vi "Teleop.vi"(10 "Match Info":T1={"Autonomous Elapsed Seconds"=0.0, "TeleOp Elapsed Seconds"=0.0, "Disabled Elapsed Seconds"=0.0, "Visited Autonomous"=FALSE, "Visited TeleOp"=FALSE, "Visited Disabled"=FALSE, "Autonomous Settings"={"Autonomous Style"=enum."Independent", "VI Refnum"=refnum}}, 11 "Call Context":T2) -> ()   [LabVIEW 2013]
doc: "This VI is called for each TeleOp packet received from the DS where the robot is not disabled. It is often used to read from the joysticks and update I/O or to update setpoints for timed control loops. It should complete and return within 20 milliseconds or it may miss DS packets."
uses:
  <vilib>/Rock Robotics/WPI/DriverStation/WPI_DriverStationDerivedRobotMode.ctl
  <vilib>/Rock Robotics/WPI/DriverStation/WPI_DriverStationMatch Info.ctl
  Robot Global Data.vi
  <vilib>/Rock Robotics/WPI/Joystick/WPI_JoystickGetSetRefNum.vi
panel:
  in  "HarvSpeed":dbl=0.5
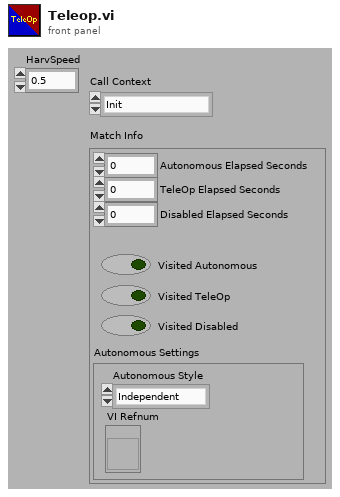
[diagram p1: front panel]
types:
  T1 = typedef "WPI_DriverStationMatch Info.ctl" = cluster{"Autonomous Elapsed Seconds":dbl, "TeleOp Elapsed Seconds":dbl, "Disabled Elapsed Seconds":dbl, "Visited Autonomous":bool, "Visited TeleOp":bool, "Visited Disabled":bool, "Autonomous Settings":cluster{"Autonomous Style":enum16{"Iterative", "Independent"}, "VI Refnum":refnum<vi>}}
  T2 = typedef "WPI_DriverStationDerivedRobotMode.ctl" = enum16{"Init", "Execute", "Stop"}
  T3 = typedef "WPI_JoystickDevRef.ctl" = cluster{"Device":T4}
  T4 = typedef "WPI_JoystickDeviceEnum.ctl" = enum16{"USB 1", "USB 2", "USB 3", "USB 4", "Kinect 1", "Kinect 2"}
  T5 = cluster{"axis 1 (x)":dbl, "axis 2 (y)":dbl, "axis 3 (throttle)":dbl, "axis 4":dbl, "axis 5":dbl, "axis 6":dbl}
  T6 = typedef "WPI_MotorControlDeviceRef.ctl" = cluster{"DeviceStatus":errorcluster, "Type":enum16{"PWM", "CAN"}, "PWM":cluster{"Digital Module":T7, "PWM Channel":T8, "DeadBand":T9}, "CAN":cluster{"Device Number":u8, "Control Mode":T10, "Semaphore":T11, "Max Vout":dbl}, "Invert":bool, "TransformRef":T12, "InvTransformRef":T12}
  T7 = typedef "FPGA_TypedefDigitalModule.ctl" = enum16{"Digital Module 1", "Digital Module 2"}
  T8 = typedef "FPGA_DIOPWMChannel.ctl" = enum8{"PWM 1", "PWM 2", "PWM 3", "PWM 4", "PWM 5", "PWM 6", "PWM 7", "PWM 8", "PWM 9", "PWM 10", "Invalid"}
  T9 = typedef "WPI_PWMDeadband.ctl" = cluster{"Name":string, "maxPositivePwm":i32, "minPositivePwm":i32, "centerPwm":i32, "maxNegativePwm":i32, "minNegativePwm":i32, "angularRange":u16}
  T10 = typedef "WPI_CANJaguar_ControlMode.ctl" = enum8{"Percent VBus", "Current", "Speed", "Position", "Voltage"}
  T11 = typedef "Semaphore RefNum" = refnum<k1>
  T12 = typedef "WPI_PWMTransform_ConPane.ctl" = refnum<vi>
  T13 = cluster{"Driver Station Digital Input (1-8)[0]":bool, "Driver Station Digital Input (1-8)[1]":bool, "Driver Station Digital Input (1-8)[2]":bool, "Driver Station Digital Input (1-8)[3]":bool, "Driver Station Digital Input (1-8)[4]":bool, "Driver Station Digital Input (1-8)[5]":bool, "Driver Station Digital Input (1-8)[6]":bool, "Driver Station Digital Input (1-8)[7]":bool, "Driver Station Digital Input (1-8)[8]":bool}
  T14 = typedef "WPI_JoystickButtonState.ctl" = cluster{"Button 1":bool, "Button 2":bool, "Button 3":bool, "Button 4":bool, "Button 5":bool, "Button 6":bool, "Button 7":bool, "Button 8":bool, "Button 9":bool, "Button 10":bool, "Button 11":bool, "Button 12":bool}
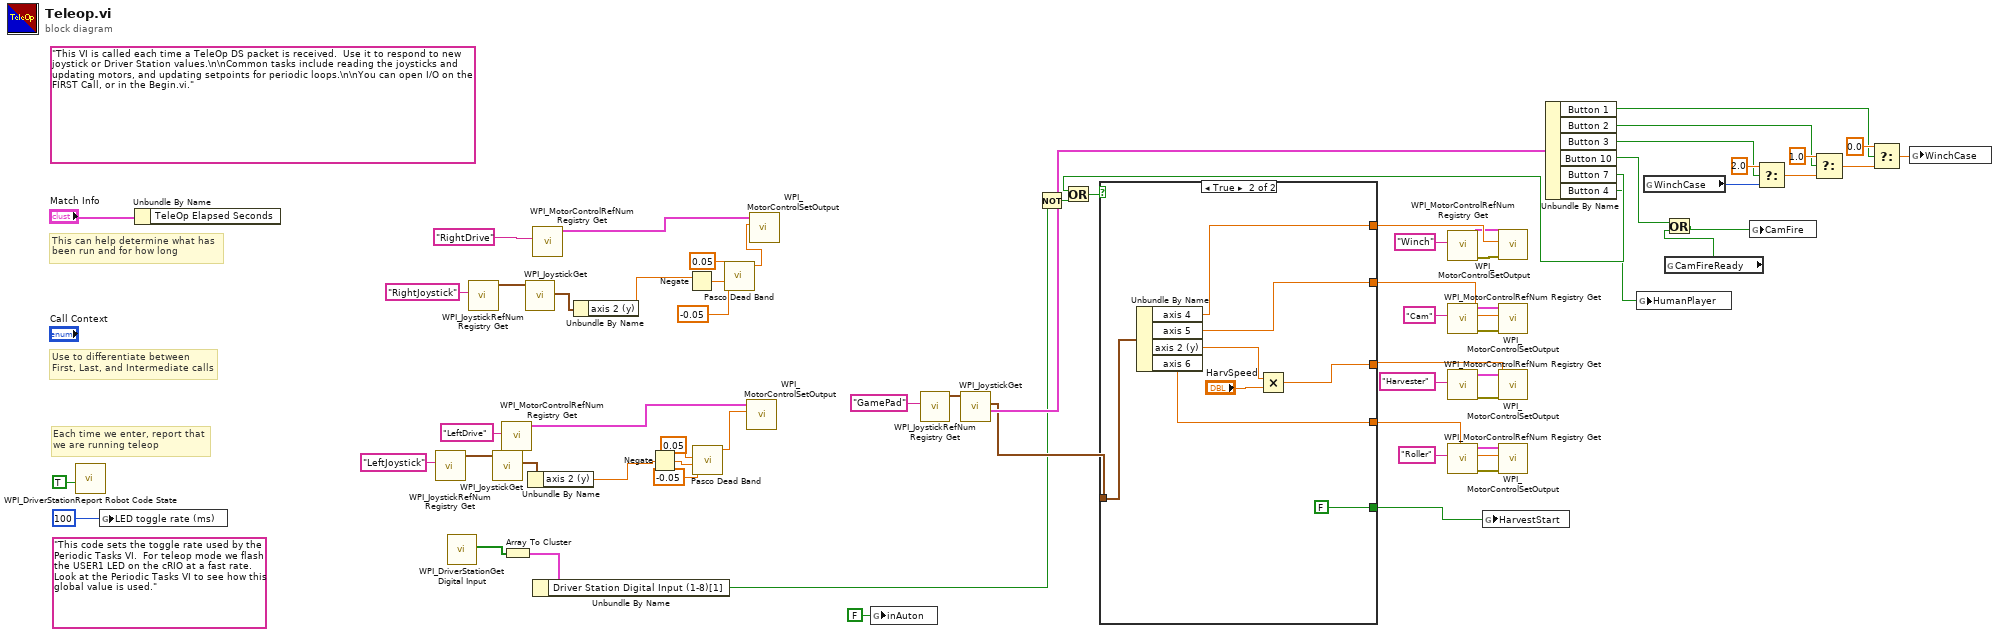
[diagram p0: block diagram]
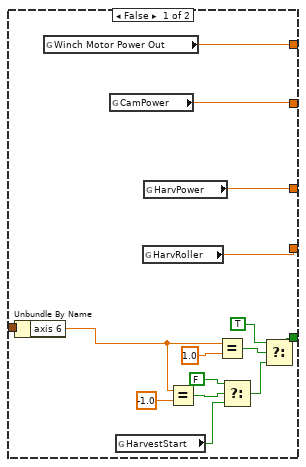
[diagram p2: hidden frame]
diagram:
  (unwired) "This code sets the toggle rate used by the Periodic Tasks VI.  For teleop mode we flash the USER1 LED on the cRIO at a fast rate.  Look at the Periodic Tasks VI to see how this global value is used."
  (unwired) "This VI is called each time a TeleOp DS packet is received.  Use it to respond to new joystick or Driver Station values.\n\nCommon tasks include reading the joysticks and updating motors, and updating setpoints for periodic loops.\n\nYou can open I/O on the FIRST Call, or in the Begin.vi."
  # "Each time we enter, report that\nwe are running teleop"
  # "Use to differentiate between\nFirst, Last, and Intermediate calls"
  # "This can help determine what has\nbeen run and for how long"
  n1 = call <vilib>:"WPI_DriverStationReport Robot Code State.vi"("TeleOp"=TRUE ("Autonomous")) -> ()  [unwired: 10 in, 1 out]
  n2 = global write "Robot Global Data.vi" "LED toggle rate (ms)"(u32 100 ("LED ms toggle rate")) -> ()
  n3 = Unbundle By Name("Match Info") -> ()  [unwired: 1 out]
  n4 = call <vilib>:"WPI_JoystickRefNum Registry Get.vi"("refnum name"="LeftJoystick") -> ("JoystickDevRef"=w54:T3)  [unwired: 9 in, 1 out]
  n5 = call <vilib>:"WPI_DriverStationGet Digital Input.vi"() -> ("Driver Station Digital Input (1-8)"=w9:bool[])  [unwired: 11 in]
  n6 = call <vilib>:"WPI_JoystickRefNum Registry Get.vi"("refnum name"="RightJoystick") -> ("JoystickDevRef"=w59:T3)  [unwired: 9 in, 1 out]
  n7 = call <vilib>:"WPI_JoystickGet.vi"("JoystickDevRef"=w54) -> ("Axes"=w53:T5)  [unwired: 4 in, 2 out]
  n8 = call <vilib>:"WPI_MotorControlRefNum Registry Get.vi"("refnum name"="LeftDrive") -> ("MotorControlDevRef"=w57:T6)  [unwired: 9 in, 1 out]
  n9 = Array To Cluster(array=w9) -> (cluster=w8:T13)
  n10 = call <vilib>:"WPI_JoystickGet.vi"("JoystickDevRef"=w59) -> ("Axes"=w58:T5)  [unwired: 4 in, 2 out]
  n11 = Unbundle By Name(w53) -> ("axis 2 (y)"=w52:dbl)
  n12 = call <vilib>:"WPI_MotorControlRefNum Registry Get.vi"("refnum name"="RightDrive") -> ("MotorControlDevRef"=w62:T6)  [unwired: 9 in, 1 out]
  n13 = Unbundle By Name(w8) -> ("Driver Station Digital Input (1-8)[1]"=w7:bool)
  n14 = Unbundle By Name(w58) -> ("axis 2 (y)"=w51:dbl)
  n15 = Negate(x=w52) -> (-x=w46:dbl)
  n16 = Negate(x=w51) -> (-x=w50:dbl)
  n17 = call "Pasco Dead Band.vi"("lower limit"=-0.05, "PWM Power"=w46, "upper limit"=0.05) -> ("PWM Power"=w43:dbl)  [unwired: 7 in, 1 out]
  n18 = call "Pasco Dead Band.vi"("lower limit"=-0.05, "PWM Power"=w50, "upper limit"=0.05) -> ("PWM Power"=w49:dbl)  [unwired: 7 in, 1 out]
  n19 = call <vilib>:"WPI_MotorControlSetOutput.vi"("Output"=w43, "MotorControlDevRef"=w57) -> ()  [unwired: 7 in, 3 out]
  n20 = call <vilib>:"WPI_MotorControlSetOutput.vi"("Output"=w49, "MotorControlDevRef"=w62) -> ()  [unwired: 7 in, 3 out]
  n21 = global write "Robot Global Data.vi" "inAuton"(FALSE ("inAuton")) -> ()
  n22 = call <vilib>:"WPI_JoystickRefNum Registry Get.vi"("refnum name"="GamePad") -> ("JoystickDevRef"=w41:T3)  [unwired: 9 in, 1 out]
  n23 = call <vilib>:"WPI_JoystickGet.vi"("JoystickDevRef"=w41) -> ("Buttons"=w14:T14, "Axes"=w13:T5)  [unwired: 4 in, 1 out]
  n24 = Not(x=w7) -> (.not. x?=w6:bool)
  n25 = call <vilib>:"WPI_MotorControlRefNum Registry Get.vi"("refnum name"="Winch") -> ("error out"=w32:errorcluster, "MotorControlDevRef"=w26:T6)  [unwired: 9 in]
  n26 = call <vilib>:"WPI_MotorControlRefNum Registry Get.vi"("refnum name"="Cam") -> ("error out"=w31:errorcluster, "MotorControlDevRef"=w30:T6)  [unwired: 9 in]
  n27 = call <vilib>:"WPI_MotorControlRefNum Registry Get.vi"("refnum name"="Harvester") -> ("error out"=w36:errorcluster, "MotorControlDevRef"=w35:T6)  [unwired: 9 in]
  n28 = call <vilib>:"WPI_MotorControlRefNum Registry Get.vi"("refnum name"="Roller") -> ("error out"=w38:errorcluster, "MotorControlDevRef"=w39:T6)  [unwired: 9 in]
  n29 = Unbundle By Name(w14) -> ("Button 1"=w17:bool, "Button 2"=w18:bool, "Button 3"=w19:bool, "Button 10"=w3:bool, "Button 7"=w10:bool, "Button 4"=w4:bool)
  n30 = Or(x=w10, y=w6) -> (x .or. y?=w11:bool)
  n31 = case shown="True" w11 {
    tunnel: [w80 w81] -> w37
    tunnel: [w79 w83] -> w33
    tunnel: w13 -> [w67 w88]
    tunnel: [w77 w87] -> w27
    tunnel: [w78 w86] -> w25
    tunnel: [w66 FALSE ("HarvestStart")] -> w12
    frame False {
      n32 = Unbundle By Name(w67) -> ("axis 6"=w75:dbl)
      n33 = global read "Robot Global Data.vi" "Winch Motor Power Out"() -> (w77:dbl)
      n34 = global read "Robot Global Data.vi" "CamPower"() -> (w78:dbl)
      n35 = global read "Robot Global Data.vi" "HarvestStart"() -> (w76:bool)
      n36 = global read "Robot Global Data.vi" "HarvRoller"() -> (w80:dbl)
      n37 = global read "Robot Global Data.vi" "HarvPower"() -> (w79:dbl)
      n38 = Equal?(x=w75, y=-1.0) -> (x = y?=w74:bool)
      n39 = Equal?(x=w75, y=1.0) -> (x = y?=w69:bool)
      n40 = Select(t=FALSE, s=w74, f=w76) -> (s? t:f=w72:bool)
      n41 = Select(t=TRUE, s=w69, f=w72) -> (s? t:f=w66:bool)
    }
    frame True {
      n42 = Unbundle By Name(w88) -> ("axis 4"=w87:dbl, "axis 5"=w86:dbl, "axis 2 (y)"=w84:dbl, "axis 6"=w81:dbl)
      n43 = Multiply(x=w84, y="HarvSpeed") -> (x*y=w83:dbl)
    }
  }
  n44 = global write "Robot Global Data.vi" "HarvestStart"(w12) -> ()
  n45 = call <vilib>:"WPI_MotorControlSetOutput.vi"("error in (no error)"=w32, "Output"=w27, "MotorControlDevRef"=w26) -> ()  [unwired: 6 in, 3 out]
  n46 = call <vilib>:"WPI_MotorControlSetOutput.vi"("error in (no error)"=w31, "Output"=w25, "MotorControlDevRef"=w30) -> ()  [unwired: 6 in, 3 out]
  n47 = call <vilib>:"WPI_MotorControlSetOutput.vi"("error in (no error)"=w36, "Output"=w33, "MotorControlDevRef"=w35) -> ()  [unwired: 6 in, 3 out]
  n48 = call <vilib>:"WPI_MotorControlSetOutput.vi"("error in (no error)"=w38, "Output"=w37, "MotorControlDevRef"=w39) -> ()  [unwired: 6 in, 3 out]
  n49 = global write "Robot Global Data.vi" "HumanPlayer"(w4) -> ()
  n50 = global read "Robot Global Data.vi" "WinchCase"() -> (w15:i32)
  n51 = global read "Robot Global Data.vi" "CamFireReady"() -> (w1:bool)
  n52 = Or(x=w3, y=w1) -> (x .or. y?=w2:bool)
  n53 = global write "Robot Global Data.vi" "CamFire"(w2) -> ()
  n54 = Select(t=2.0, s=w19, f=w15) -> (s? t:f=w24:dbl)
  n55 = Select(t=1.0, s=w18, f=w24) -> (s? t:f=w23:dbl)
  n56 = Select(t=0.0, s=w17, f=w23) -> (s? t:f=w16:dbl)
  n57 = global write "Robot Global Data.vi" "WinchCase"(w16) -> ()
